vi "highlightRowSelection.vi"(8 "error in (no error)":errorcluster, 10 "rowIndex":i32, 11 "ScriptEditorV2 in":refnum<class "ScriptEditorV2.lvclass">) -> (0 "error out":errorcluster, 3 "ScriptEditorV2 out":refnum<class "ScriptEditorV2.lvclass">)   [LabVIEW 2009, in "Views.lvlib" / "ScriptEditor.lvlib" / "ScriptEditorV2.lvclass"]
uses:
  ScriptEditorV2.lvclass
  ScriptEditorV2.lvclass/ScriptEditorV2.ctl
  Tools/Scripting/ScriptingEvent/ScriptEventList/ScriptEventList.lvclass
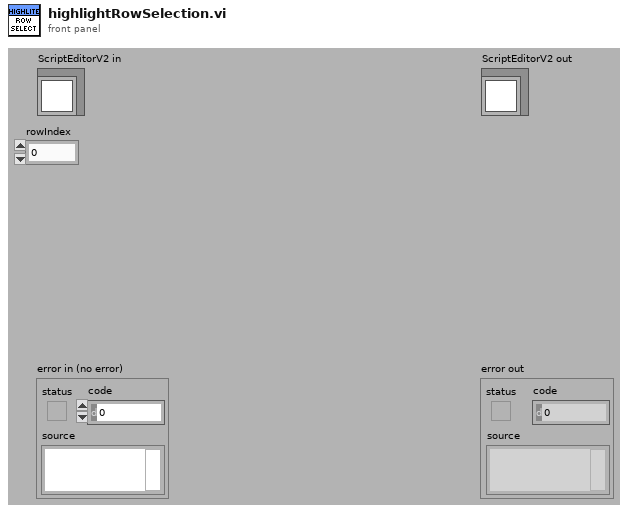
[diagram p1: front panel]
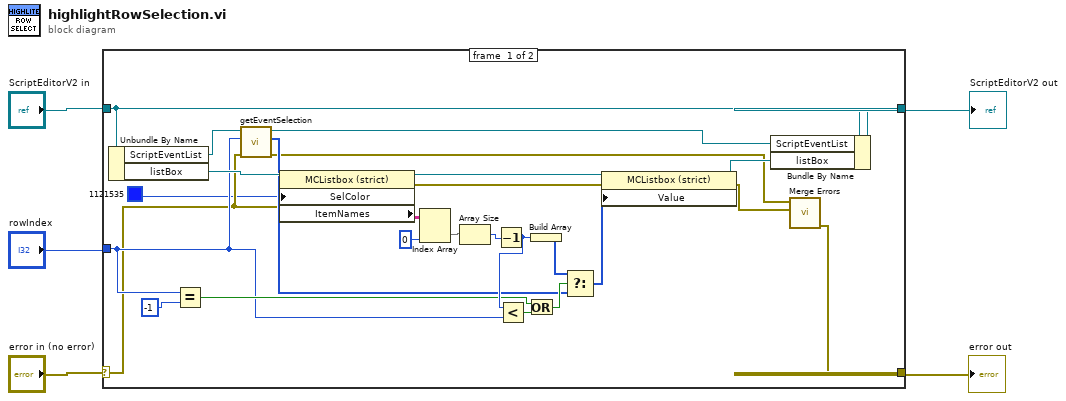
[diagram p0: block diagram]
diagram:
  n1 = case shown="No Error" "error in (no error)" {
    selector: "error in (no error)" -> [w11 w33]
    tunnel: [w7 w33] -> w4
    tunnel: [w29 w32] -> w2
    tunnel: "ScriptEditorV2 in" -> [w30 w32]
    tunnel: "rowIndex" -> [w13 _]
    frame #0 {
      n2 = Unbundle By Name(w30) -> ("ScriptEventList"=w14:refnum<class "ScriptEventList.lvclass">, "listBox"=w31:refnum<vi>)
      n3 = Equal?(x=w13, y=-1) -> (x = y?=w16:bool)
      n4 = call "getEventSelection.vi"("error in (no error)"=w11, "selectedIndex"=w13, "ScriptEventList in"=w14) -> ("error out"=w9:errorcluster, "indexArray"=w12:i32[], "ScriptEventList out"=w10:refnum<class "ScriptEventList.lvclass">)  [unwired: 6 in]
      n5 = property class="MCListbox (strict)"(reference=w31, error in=w11, "SelColor"=u32 1121535) -> (reference out=w22:refnum<vi>, error out=w20:errorcluster, "ItemNames"=w27:string[][])
      n6 = Index Array(array=w27, index (col)=0) -> (element=w25:string[])  [unwired: 1 in]
      n7 = Array Size(array=w25) -> (size(s)=w24:i32)
      n8 = Decrement(x=w24) -> (x-1=w17:i32)
      n9 = Less?(x=w17, y=w13) -> (x < y?=w18:bool)
      n10 = Or(x=w16, y=w18) -> (x .or. y?=w15:bool)
      n11 = Build Array(w17) -> (w23:i32[])
      n12 = Select(t=w23, s=w15, f=w12) -> (s? t:f=w21:i32[])
      n13 = property class="MCListbox (strict)"(reference=w22, error in=w20, "Value"=w21) -> (reference out=w19:refnum<vi>, error out=w8:errorcluster)
      n14 = Bundle By Name(cluster=w30, "ScriptEventList"=w10, "listBox"=w19) -> (w29:refnum<class "ScriptEditorV2.lvclass">)
      n15 = call <vilib>:"Merge Errors.vi"("error in 2 (no error)"=w8, "error in 1 (no error)"=w9) -> ("error out"=w7:errorcluster)  [unwired: 5 in]
    }
    frame #1 {
    }
  }
  "error out" <- w4
  "ScriptEditorV2 out" <- w2
